vi "readFromXMLElevation.vi"(8 "error in (no error)":errorcluster, 10 "XML in":string="<Elevation>\n  <degreesAlt>90.10</degreesAlt>\n  <minutesArc>80.10</minutesArc>\n  <secondsArc>70.10</secondsArc>\n</Elevation>") -> (0 "error out":errorcluster)   [LabVIEW 2012]
uses:
  <userlib>/Common/UnitsAndXML/FlattenItemWithUnitToXML/FlattenPlaneAngleToXML/PlaneAngleUnit.ctl
  <userlib>/Common/UnitsAndXML/UnitsAndXML.lvlib
  <userlib>/Common/XML/XMLParser/XMLParser.lvclass
panel:
  out "attributeData":T1(array[cluster])
  in  "secondsArc 2":dbl[unit]=0.0003398543904577847
  in  "minutesArc 2":dbl[unit]=0.023300145514124296
  in  "degreesAlt 2":dbl[unit]=1.5725416560468908
  out "Element out":refnum<class "XMLParser.lvclass">
  in  "Element in":refnum<class "XMLParser.lvclass">=refnum
  out "secondsArc":dbl[unit]=0.0003398543904577847
  out "minutesArc":dbl[unit]=0.023300145514124296
  out "degreesAlt":dbl[unit]=1.5725416560468908
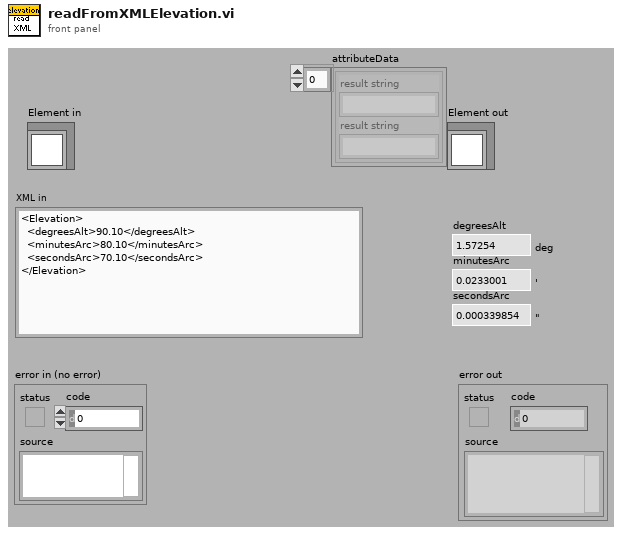
[diagram p1: front panel]
types:
  T1 = cluster{"result string":string, "result string":string}[]
  T2 = typedef "UnitsAndXML.lvlib/PlaneAngleUnit.ctl" = enum16{"rad", "deg", "'", "\""}
  T3 = typedef "AttributeElements.ctl" = cluster{"attributeType":string, "attributeValue":string}
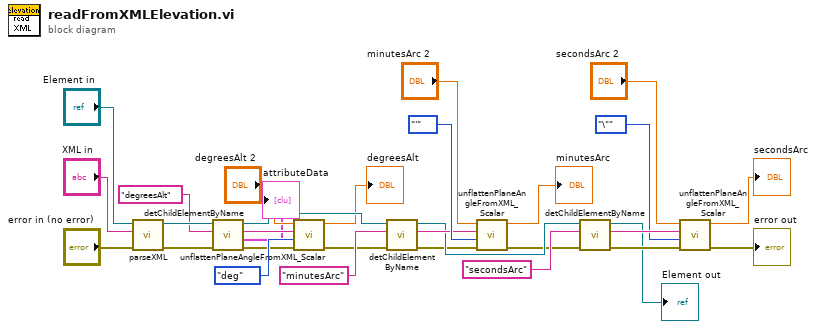
[diagram p0: block diagram]
diagram:
  n1 = call <userlib>:"parseXML.vi"("error in (no error)"="error in (no error)", "XMLString in"="XML in", "Element in"="Element in") -> ("error out"=w22:errorcluster, "Element out"=w27:refnum<class "XMLParser.lvclass">)  [unwired: 7 in]
  n2 = call <userlib>:"detChildElementByName.vi"("error in (no error)"=w22, "childName"="degreesAlt" ("ChildName"), "Element in"=w27) -> ("error out"=w23:errorcluster, "childAttributes"=→"attributeData":T3[], "childXML"=w25:string, "Element out"=w21:refnum<class "XMLParser.lvclass">)  [unwired: 5 in]
  n3 = call <userlib>:"unflattenPlaneAngleFromXML_Scalar.vi"("error in (no error)"=w23, "planeAngleUnitInXML"=PlaneAngleUnit."deg", "xmlString"=w25, "planeAngleForType"="degreesAlt 2") -> ("error out"=w10:errorcluster, "planeAngle"=→"degreesAlt":dbl[unit])  [unwired: 6 in]
  n4 = call <userlib>:"detChildElementByName.vi"("error in (no error)"=w10, "childName"="minutesArc" ("ChildName"), "Element in"=w21) -> ("error out"=w9:errorcluster, "childXML"=w17:string, "Element out"=w16:refnum<class "XMLParser.lvclass">)  [unwired: 5 in, 1 out]
  n5 = call <userlib>:"unflattenPlaneAngleFromXML_Scalar.vi"("error in (no error)"=w9, "planeAngleUnitInXML"=PlaneAngleUnit."'", "xmlString"=w17, "planeAngleForType"="minutesArc 2") -> ("error out"=w8:errorcluster, "planeAngle"=→"minutesArc":dbl[unit])  [unwired: 6 in]
  n6 = call <userlib>:"detChildElementByName.vi"("error in (no error)"=w8, "childName"="secondsArc" ("ChildName"), "Element in"=w16) -> ("error out"=w7:errorcluster, "childXML"=w14:string, "Element out"=→"Element out":refnum<class "XMLParser.lvclass">)  [unwired: 5 in, 1 out]
  n7 = call <userlib>:"unflattenPlaneAngleFromXML_Scalar.vi"("error in (no error)"=w7, "planeAngleUnitInXML"=PlaneAngleUnit."\"", "xmlString"=w14, "planeAngleForType"="secondsArc 2") -> ("error out"=→"error out":errorcluster, "planeAngle"=→"secondsArc":dbl[unit])  [unwired: 6 in]
